vi "8-Axis Roadshow Demo WPC-IPAD.vi"() -> ()   [LabVIEW 2014]
uses:
  Typedef/Typedef_Motor_Message.ctl
  EMC API/EMC_Typedef_Motor_Parameters.ctl
  Functional_Global/Typedef_Message_Queue_Action.ctl
  Functional_Global/Typedef_FPGA_Interface_Action.ctl
  Globals/Global Stop.vi
  Globals/Default Motor Parameters.vi
  <vilib>/Motion/Express/_s/nimc.ex.clearFaults.clearFaults.axis.vi
  <vilib>/Motion/Express/_s/nimc.ex.power.power.axis.vi
  <vilib>/Motion/Express/_s/nimc.ex.resetPosition.resetPosition.axis.vi
  <vilib>/Motion/Express/_s/nimc.ex.read.readTrajectoryData.axis.vi
  <vilib>/Motion/BlockNode/FB.NIMotion.xnode
  support/Message Queue/Message Queue.lvlib
  <vilib>/NI_Real-Time Target Support.lvlib
panel:
  in  "Mode":u16
  in  "# whole revs":dbl=3.0 format="%#_13g"
  in  "Stop all motors":bool
  in  "Max delay (ms)":u32=1000
  in  "Motion Parameters (Min)":T1={"position"=-2000.0, "velocity"=500.0, "acceleration"=5000.0, "deceleration"=5000.0, "accel. jerk"=80000.0, "decel. jerk"=80000.0}
  in  "Motion Parameters (Max)":T1={"position"=2000.0, "velocity"=1500.0, "acceleration"=10000.0, "deceleration"=10000.0, "accel. jerk"=100000.0, "decel. jerk"=100000.0}
  in  "Command Array":string[](array[string])=["ABS Pos Move", "REL Pos Move", "Velocity Move"]
  out "Command":T2={"Axis"="Axis 8", "Motion Parameters"={"position"=0.0, "velocity"=0.0, "acceleration"=0.0, "deceleration"=0.0, "accel. jerk"=0.0, "decel. jerk"=0.0}}
  out "Message":string="Stop"
  out "# elements in queue":i32=9
  out "error out":errorcluster
  out "Axis Positions":T3(graph)={"[0]"=16540.00000000011, "[1]"=7939.956878279383, "[2]"=-7459.9999999999345, "[3]"=-3059.9999999999545, "[4]"=-26059.999999999975, "[5]"=22740.000000000004, "[6]"=3139.9999999999973, "[7]"=11139.999999999998}
  out "Axis Velocities":T3(graph)
  out "Array":dbl[](array[knob])=[140.00000000010914, 139.9568782793831, 140.00000000006548, 140.00000000004547, 140.00000000002547, 140.00000000000364, 139.99999999999727, 139.99999999999818] scale=0.0..200.0
  in  "stop":bool
  # "This example demonstrates how to set up an multi-axis SW architecture using SoftMotion.  You can have state machines that \"produce\" the motion commands, and the consumer will then digest them one at a time.\n\nIn this example, 3 producer loops generate random motion commands at random times (within 1000ms each iteration.) This VI is also meant as a stress test to see if the SM engine is robust enough for complex sequences of motion commands."
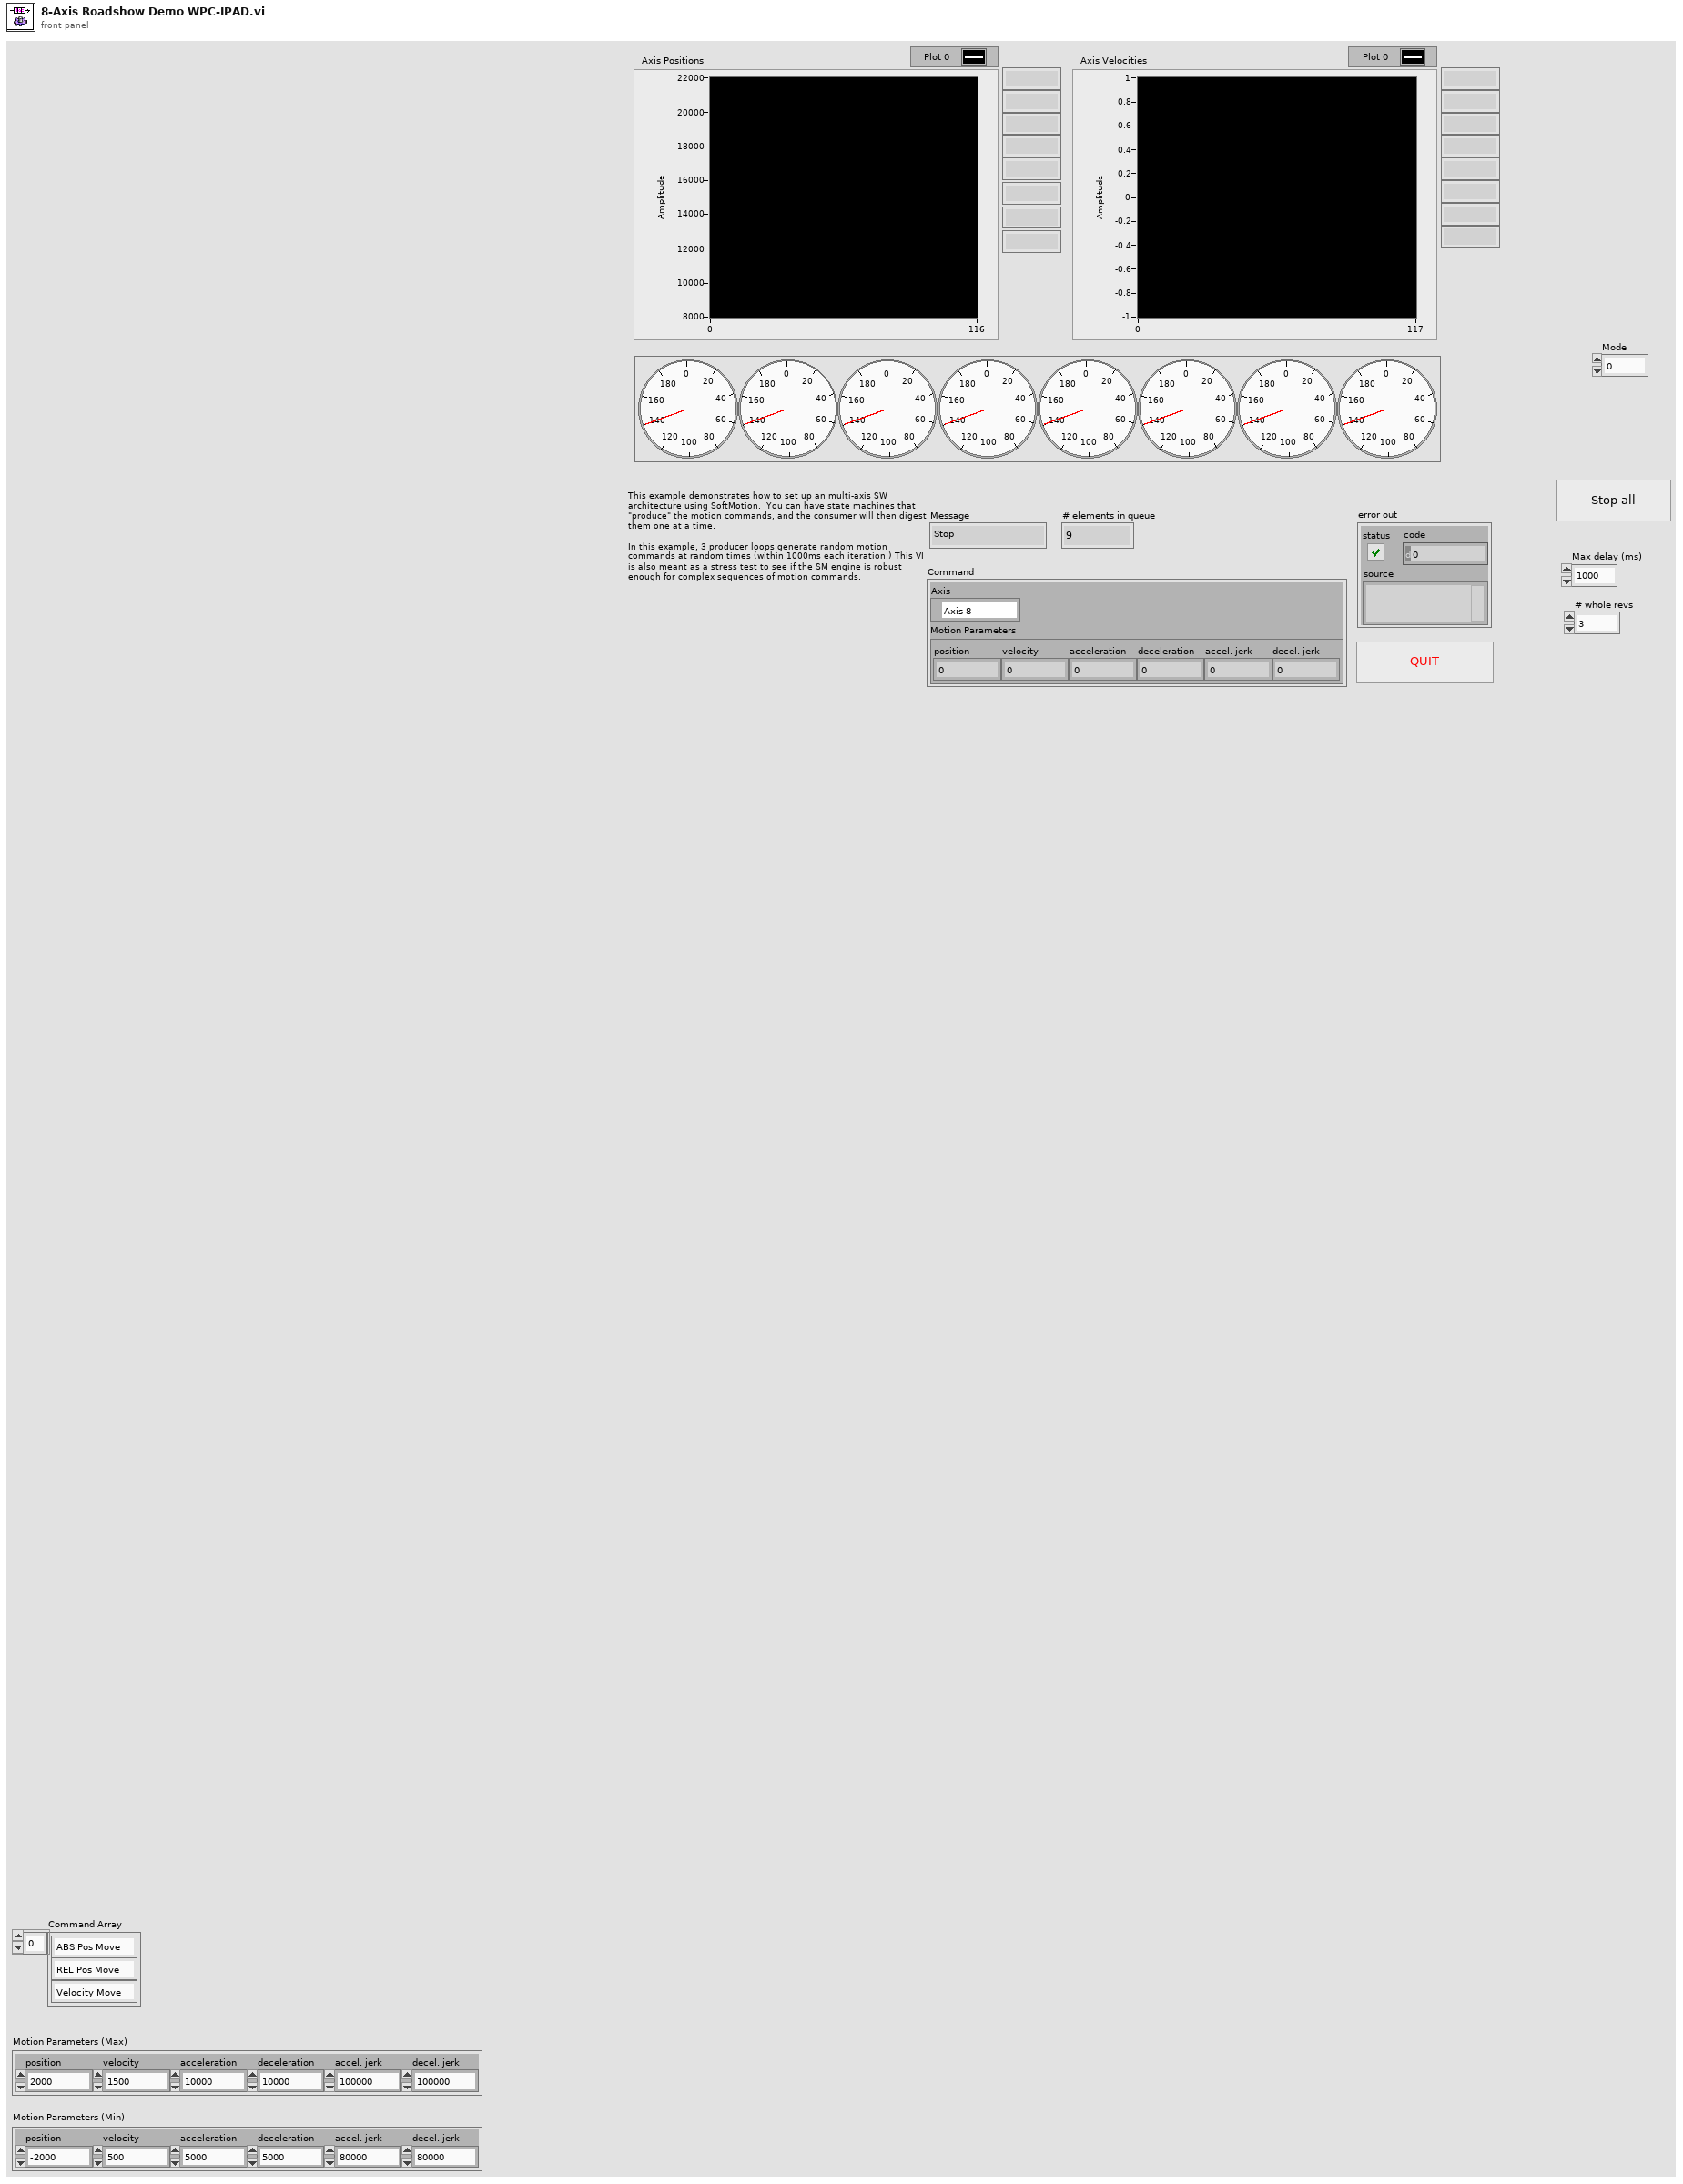
[diagram p1: front panel]
types:
  T1 = typedef "EMC_Typedef_Motor_Parameters.ctl" = cluster{"position":dbl, "velocity":dbl, "acceleration":dbl, "deceleration":dbl, "accel. jerk":dbl, "decel. jerk":dbl}
  T2 = typedef "Typedef_Motor_Message.ctl" = cluster{"Axis":refnum<k21>, "Motion Parameters":T1}
  T3 = cluster{"[0]":dbl, "[1]":dbl, "[2]":dbl, "[3]":dbl, "[4]":dbl, "[5]":dbl, "[6]":dbl, "[7]":dbl}
  T4 = typedef "Typedef_Message_Queue_Action.ctl" = enum16{"Init MQueue", "Get MQueue Ref", "Close MQueue"}
  T5 = typedef "Typedef_FPGA_Interface_Action.ctl" = enum16{"Initialize FPGA", "Get FPGA Reference", "Close FPGA"}
  T6 = typedef "Message Queue.lvlib/Message Cluster.ctl" = cluster{"Message":string, "Message Data":variant}
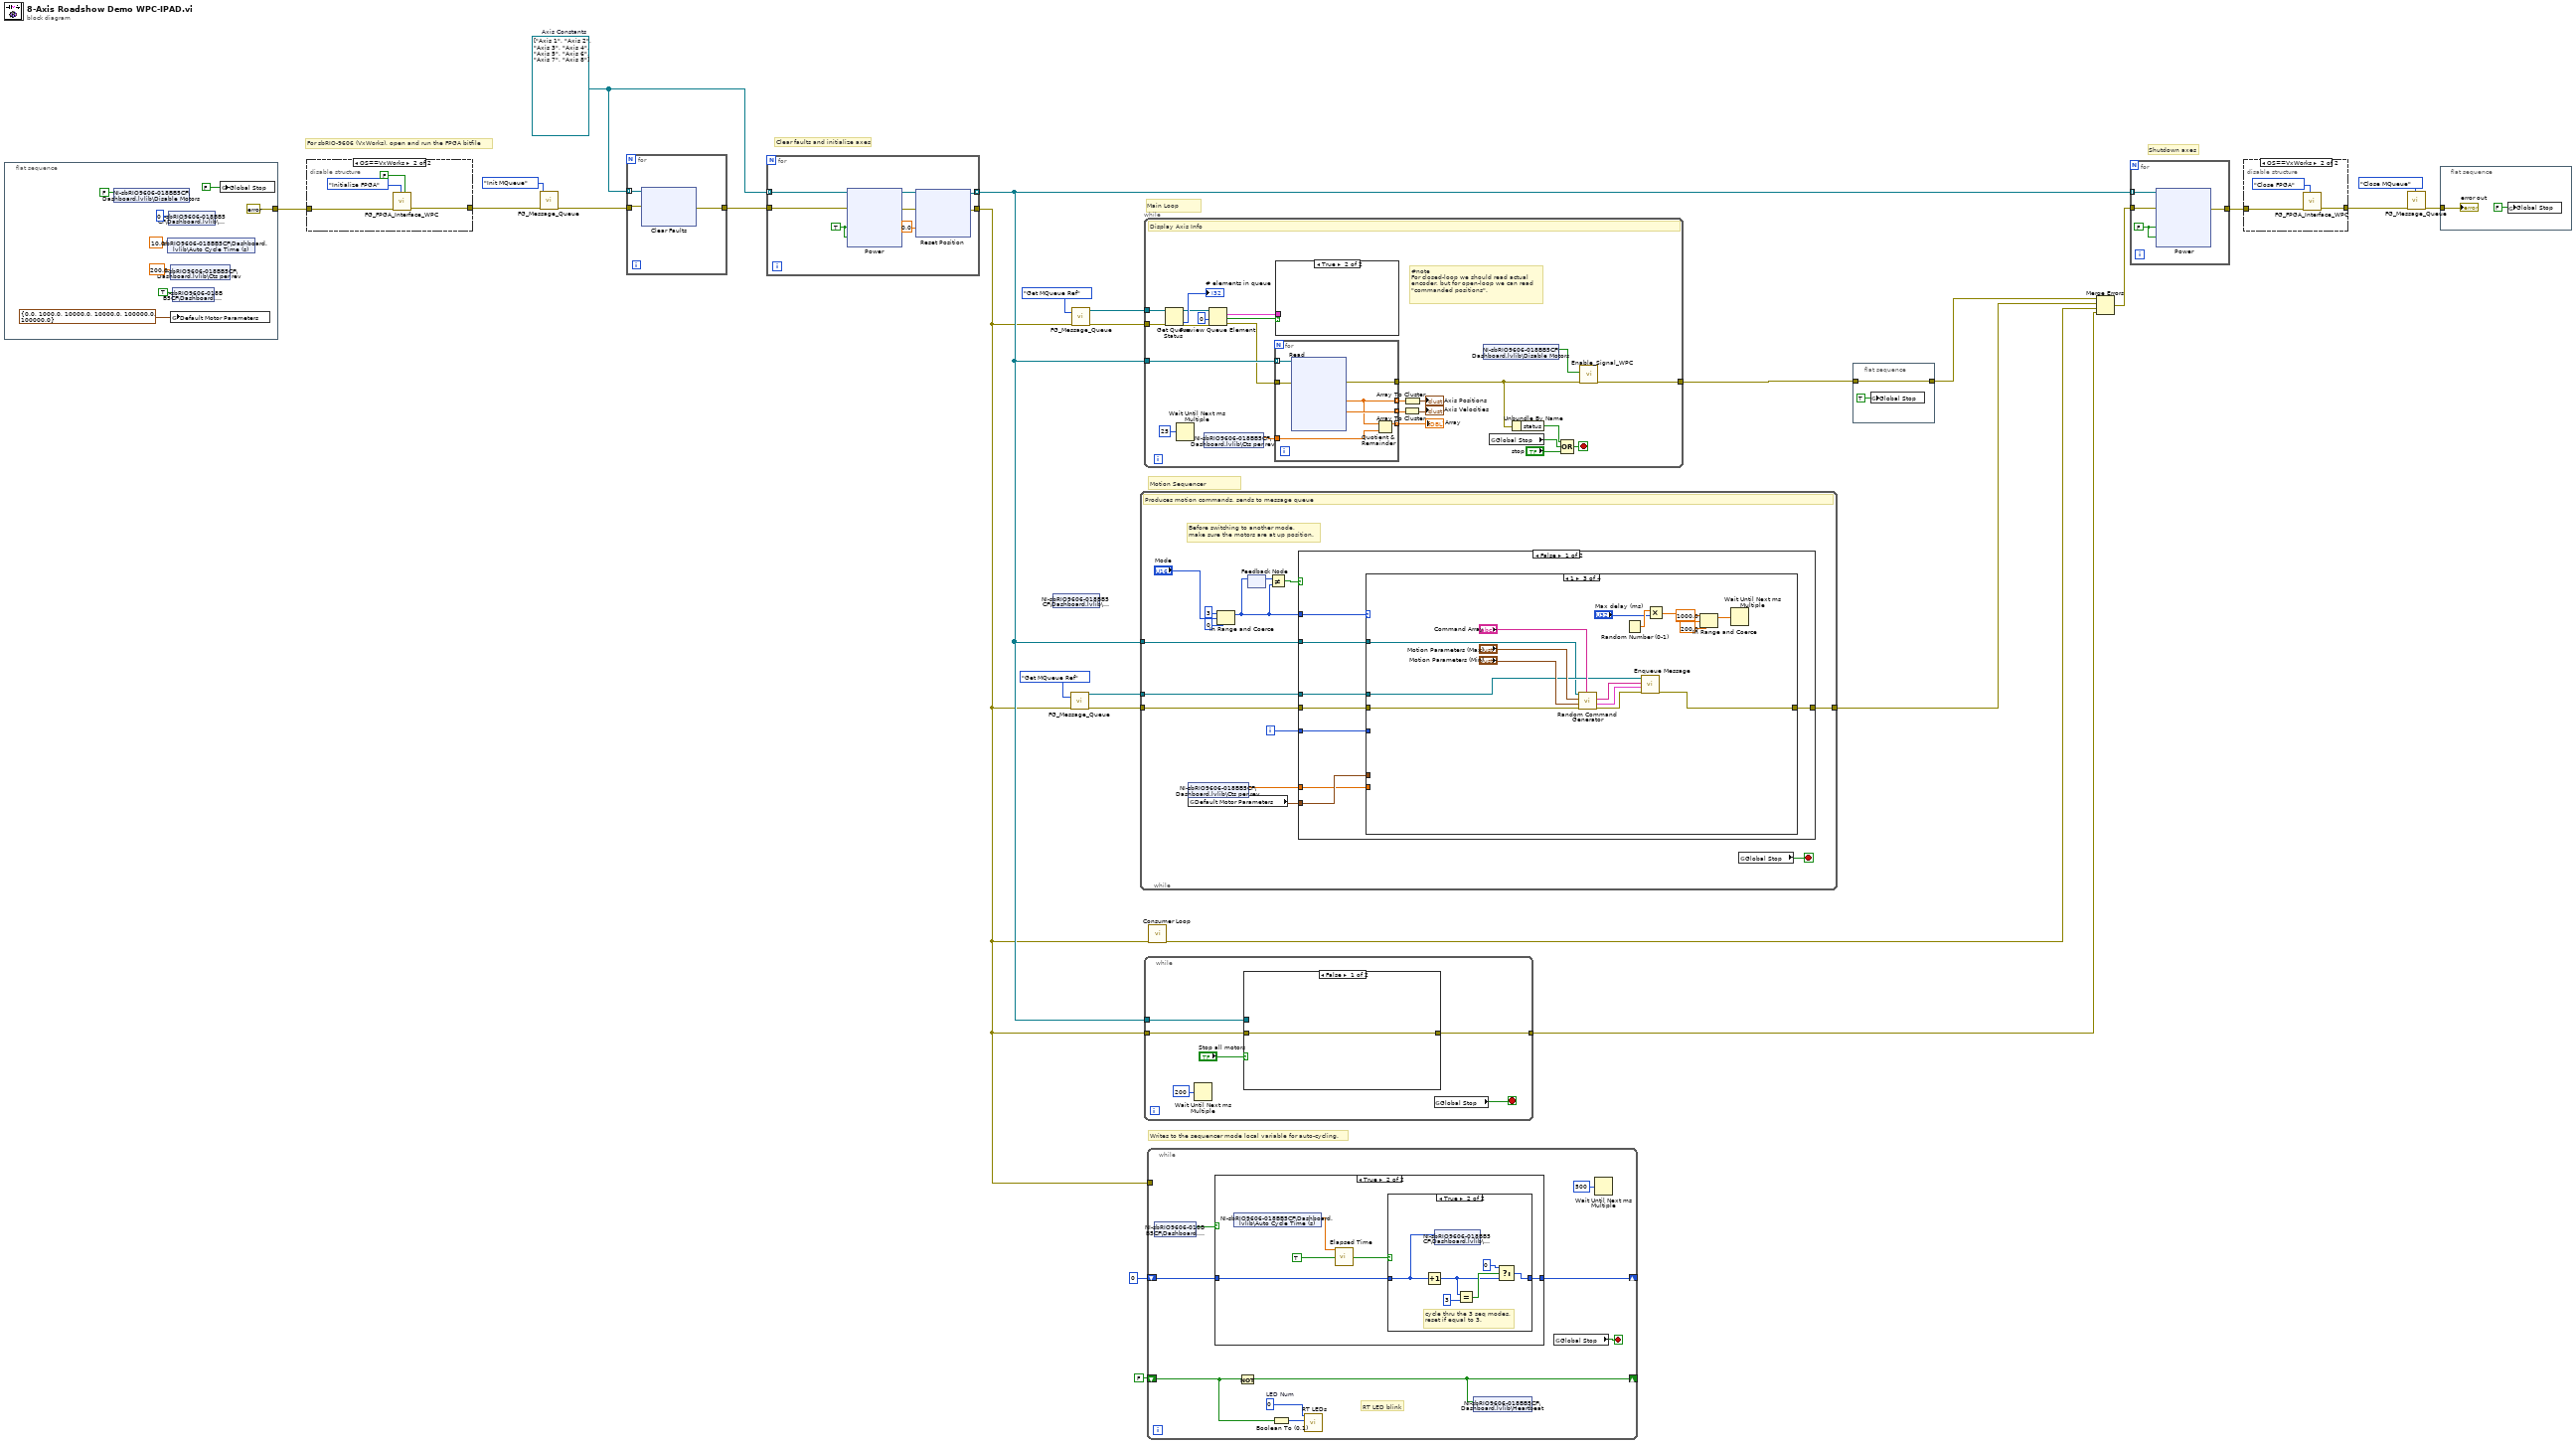
[diagram p0: block diagram]
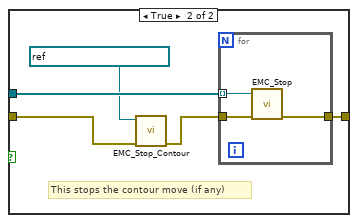
[diagram p4: hidden frame]
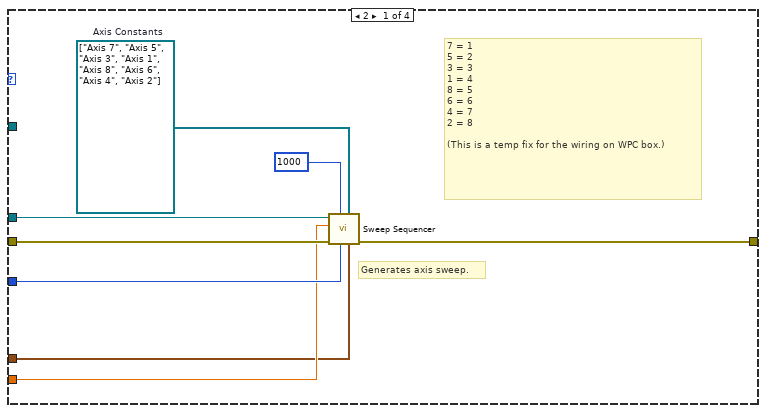
[diagram p5: hidden frame]
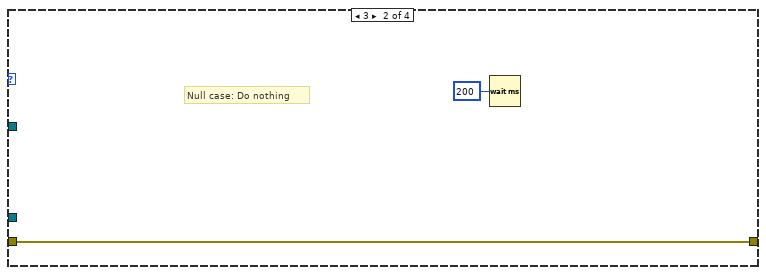
[diagram p6: hidden frame]
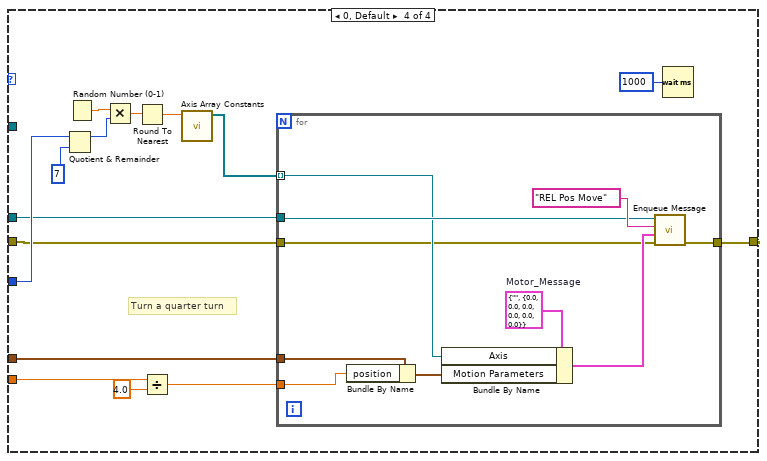
[diagram p7: hidden frame]
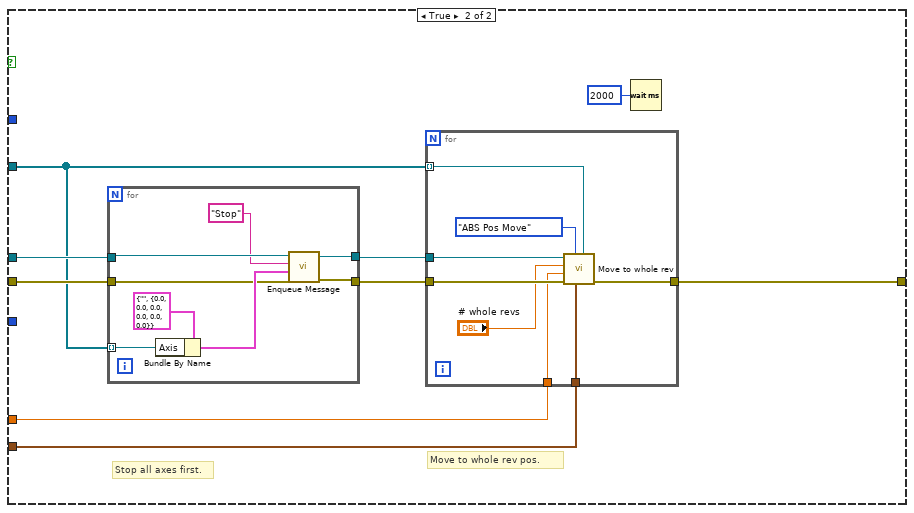
[diagram p8: hidden frame]
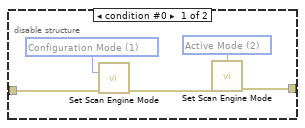
[diagram p10: hidden frame]
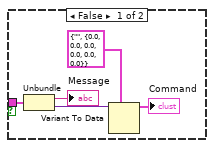
[diagram p11: hidden frame]
diagram:
  w1 = refnum<k21>[] ["Axis 1", "Axis 2", "Axis 3", "Axis 4", "Axis 5", "Axis 6", "Axis 7", "Axis 8"]  # Axis Constants
  # "Writes to the sequencer mode local variable for auto-cycling."
  # "Motion Sequencer"
  # "For sbRIO-9606 (VxWorks), open and run the FPGA bitfile"
  # "Shutdown axes"
  # "Main Loop"
  # "Clear faults and initialize axes"
  n1 = flat-sequence {
    tunnel: [errorcluster {"status"=FALSE, "code"=0, "source"=""} ("error in (no error)")] -> w26
    frame #0 {
      n2 = shared-variable "NI-sbRIO9606-018BB5CF\\Dashboard.lvlib\\Disable Motors"(FALSE ("Disable Motors")) -> ()  [unwired: 1 in, 1 out]
      n3 = shared-variable "NI-sbRIO9606-018BB5CF\\Dashboard.lvlib\\Auto Cycle Time (s)"(10.0 ("Auto Cycle Time (s)")) -> ()  [unwired: 1 in, 1 out]
      n4 = shared-variable "NI-sbRIO9606-018BB5CF\\Dashboard.lvlib\\Mode"(u16 0 ("Mode")) -> ()  [unwired: 1 in, 1 out]
      n5 = shared-variable "NI-sbRIO9606-018BB5CF\\Dashboard.lvlib\\Cts per rev"(200.0 ("Cts per rev")) -> ()  [unwired: 1 in, 1 out]
      n6 = global write "Default Motor Parameters.vi" "Default Motor Parameters"(T1 {"position"=0.0, "velocity"=1000.0, "acceleration"=10000.0, "deceleration"=10000.0, "accel. jerk"=100000.0, "decel. jerk"=100000.0} ("Default Motor Parameters")) -> ()
      n7 = shared-variable "NI-sbRIO9606-018BB5CF\\Dashboard.lvlib\\Auto"(TRUE ("Auto")) -> ()  [unwired: 1 in, 1 out]
      n8 = global write "Global Stop.vi" "Global Stop"(FALSE ("stop")) -> ()
    }
  }
  n9 = disable-structure shown="OS==VxWorks" {
    disable-tunnel: [w39 w41] -> w22
    disable-tunnel: w26 -> [w38 w42]
    frame condition #0 {
      w35 = 1 items=["Configuration Mode"=1, "Active Mode"=2] ("mode (Active Mode)")
      w36 = 2 items=["Configuration Mode"=1, "Active Mode"=2] ("mode (Active Mode)")
      n10 = call <vilib>:"Set Scan Engine Mode.vi"("mode (Active Mode)"=w35, "error in (no error)"=w38) -> ("error out"=w37:errorcluster)  [unwired: 13 in]
      n11 = call <vilib>:"Set Scan Engine Mode.vi"("mode (Active Mode)"=w36, "error in (no error)"=w37) -> ("error out"=w39:errorcluster)  [unwired: 13 in]
    }
    frame condition #1 (active) {
      n12 = call "FG_FPGA_Interface_WPC.vi"("Invert Dir?"=FALSE, "Action"=Typedef_FPGA_Interface_Action."Initialize FPGA", "error in"=w42) -> ("error out"=w41:errorcluster)  [unwired: 7 in, 1 out]
    }
  }
  n13 = call "FG_Message_Queue.vi"("Action"=Typedef_Message_Queue_Action."Init MQueue", "error in"=w22) -> ("error out"=w3:errorcluster)  [unwired: 8 in, 1 out]
  n14 = for {
    tunnel: w3 -> [w46]
    tunnel: [w45] -> w2
    tunnel: w1 -> [w44] mode=indexing
    n15 = xnode ("Clear Faults")("resource"=w44, "error in"=w46) -> ("error out"=w45:errorcluster)  [unwired: 1 out]
  }
  n16 = for {
    tunnel: [w55] -> w6
    tunnel: [w53] -> w8 mode=indexing
    tunnel: w2 -> [w52]
    tunnel: w1 -> [w51] mode=indexing
    w58 = TRUE ("enable axis")
    n17 = xnode ("Power")("enable axis"=w58, "enable drive"=w58, "resource"=w51, "error in"=w52) -> ("resource out"=w54:refnum<k21>, "error out"=w56:errorcluster)
    n18 = xnode ("Reset Position")("position"=0.0, "resource"=w54, "error in"=w56) -> ("resource out"=w53:refnum<k21>, "error out"=w55:errorcluster)
  }
  n19 = shared-variable "NI-sbRIO9606-018BB5CF\\Dashboard.lvlib\\Mode"() -> ()  [unwired: 1 in, 2 out]
  n20 = call "FG_Message_Queue.vi"("Action"=Typedef_Message_Queue_Action."Get MQueue Ref", "error in"=w6) -> ("error out"=w11:errorcluster, "Message Queue"=w10:refnum<queue>)  [unwired: 8 in]
  n21 = call "FG_Message_Queue.vi"("Action"=Typedef_Message_Queue_Action."Get MQueue Ref", "error in"=w6) -> ("error out"=w14:errorcluster, "Message Queue"=w15:refnum<queue>)  [unwired: 8 in]
  n22 = while {
    tunnel: w8 -> [w84]
    tunnel: w11 -> [w86]
    tunnel: w10 -> [w85]
    tunnel: [w82] -> w9
    i -> [w83]
    stop <- w87 stop-if-true
    # "Before switching to another mode,\nmake sure the motors are at up position."
    # "Produces motion commands, sends to message queue"
    n23 = shared-variable "NI-sbRIO9606-018BB5CF\\Dashboard.lvlib\\Cts per rev"() -> (w75:dbl)  [unwired: 1 in, 1 out]
    n24 = global read "Default Motor Parameters.vi" "Default Motor Parameters"() -> (w79:T1)
    n25 = In Range and Coerce(upper limit=u16 3, x="Mode", lower limit=u16 0) -> (coerced(x)=w76:u16)  [unwired: 1 out]
    n26 = feedback-in #1(w76) -> ()
    n27 = feedback #1() -> (w81:u16)  [unwired: 1 in]
    n28 = Not Equal?(x=w81, y=w76) -> (x != y?=w80:bool)
    n29 = case shown="False" w80 {
      tunnel: w86 -> [w95 w152]
      tunnel: w85 -> [w94 w153]
      tunnel: w84 -> [w93 w149]
      tunnel: w83 -> [w92 _]
      tunnel: [w91 w155] -> w82
      tunnel: w76 -> [w90 _]
      tunnel: w79 -> [w89 w148]
      tunnel: w75 -> [w88 w147]
      frame False {
        n30 = case shown="1" w90 {
          tunnel: w95 -> [w103 w105 w115 w134]
          tunnel: w94 -> [w101 _ w114 w132]
          tunnel: w93 -> [_ _ w113 _]
          tunnel: w92 -> [w102 _ _ w135]
          tunnel: [w100 w105 w111 w133] -> w91
          tunnel: w89 -> [w97 _ _ w127]
          tunnel: w88 -> [w98 _ _ w126]
          frame 2 {
            w96 = refnum<k21>[] ["Axis 7", "Axis 5", "Axis 3", "Axis 1", "Axis 8", "Axis 6", "Axis 4", "Axis 2"]  # Axis Constants
            # "7 = 1\n5 = 2\n3 = 3\n1 = 4\n8 = 5\n6 = 6\n4 = 7\n2 = 8\n\n(This is a temp fix for the wiring on WPC box.)"
            # "Generates axis sweep."
            n31 = call "Sweep Sequencer.vi"("Default Motor Parameters"=w97, "Axis Array"=w96, "Loop counter in"=w102, "Max delay (ms)"=u32 1000, "error in (no error)"=w103, "cts per rev"=w98, "Message Queue"=w101) -> ("error out"=w100:errorcluster)  [unwired: 4 in]
          }
          frame 3 {
            # "Null case: Do nothing"
            n32 = Wait (ms)(milliseconds to wait=u32 200) -> ()  [unwired: 1 out]
          }
          frame 1 {
            n33 = call "Random Command Generator.vi"("Command Array"="Command Array", "error in (no error)"=w115, "Motion Parameters (Min)"="Motion Parameters (Min)", "Motion Parameters (Max)"="Motion Parameters (Max)", "Axis Resources"=w113) -> ("error out"=w116:errorcluster, "Motor_Message"=w118:T2, "Command Out"=w117:string)  [unwired: 4 in]
            n34 = Random Number (0-1)() -> (number: 0 to 1=w112:dbl)
            n35 = call "Enqueue Message.vi"("error in (no error)"=w116, "Message Data"=w118, "Message"=w117, "Message Queue"=w114) -> ("error out"=w111:errorcluster)  [unwired: 6 in, 1 out]
            n36 = Multiply(x=w112, y="Max delay (ms)") -> (x*y=w109:dbl)
            n37 = In Range and Coerce(upper limit=1000.0, x=w109, lower limit=200.0) -> (coerced(x)=w106:dbl)  [unwired: 1 out]
            n38 = Wait Until Next ms Multiple(millisecond multiple=w106) -> ()  [unwired: 1 out]
          }
          frame 0, Default {
            # "Turn a quarter turn"
            n39 = Quotient & Remainder(x=w135, y=7) -> (x-y*floor(x/y)=w129:i32)  [unwired: 1 out]
            n40 = Random Number (0-1)() -> (number: 0 to 1=w130:dbl)
            n41 = Multiply(x=w130, y=w129) -> (x*y=w128:dbl)
            n42 = Round To Nearest(number=w128) -> (nearest integer value=w122:dbl)
            n43 = Divide(x=w126, y=4.0) -> (x/y=w124:dbl)
            n44 = call "Axis Array Constants.vi"("Numeric"=w122) -> ("Axis Constants"=w123:refnum<k21>[])  [unwired: 10 in]
            n45 = for {
              tunnel: w123 -> [w141] mode=indexing
              tunnel: w134 -> [w140]
              tunnel: [w139] -> w133
              tunnel: w124 -> [w142]
              tunnel: w132 -> [w143]
              tunnel: w127 -> [w137]
              w146 = T2 {"Axis"="", "Motion Parameters"={"position"=0.0, "velocity"=0.0, "acceleration"=0.0, "deceleration"=0.0, "accel. jerk"=0.0, "decel. jerk"=0.0}}  # Motor_Message
              n46 = Bundle By Name(cluster=w137, "position"=w142) -> (w138:T1)
              n47 = Bundle By Name(cluster=w146, "Axis"=w141, "Motion Parameters"=w138) -> (w145:T2)
              n48 = call "Enqueue Message.vi"("error in (no error)"=w140, "Message Data"=w145, "Message"="REL Pos Move", "Message Queue"=w143) -> ("error out"=w139:errorcluster)  [unwired: 6 in, 1 out]
            }
            n49 = Wait (ms)(milliseconds to wait=u32 1000) -> ()  [unwired: 1 out]
          }
        }
      }
      frame True {
        # "Move to whole rev pos."
        # "Stop all axes first."
        n50 = for {
          tunnel: w153 -> [w163]
          tunnel: w152 -> [w157]
          tunnel: [w156] -> w151
          tunnel: [w161] -> w150
          tunnel: w149 -> [w158] mode=indexing
          n51 = Bundle By Name(cluster=T2 {"Axis"="", "Motion Parameters"={"position"=0.0, "velocity"=0.0, "acceleration"=0.0, "deceleration"=0.0, "accel. jerk"=0.0, "decel. jerk"=0.0}} ("Motor_Message"), "Axis"=w158) -> (w159:T2)
          n52 = call "Enqueue Message.vi"("error in (no error)"=w157, "Message Data"=w159, "Message"="Stop", "Message Queue"=w163) -> ("error out"=w156:errorcluster, "dup Message Queue"=w161:refnum<queue>)  [unwired: 6 in]
        }
        n53 = for {
          tunnel: w149 -> [w167] mode=indexing
          tunnel: w151 -> [w171]
          tunnel: [w170] -> w155
          tunnel: w150 -> [w169]
          tunnel: w148 -> [w166]
          tunnel: w147 -> [w165]
          n54 = call "Move to whole rev.vi"("resource in"=w167, "Default Motor Parameters"=w166, "Mode"=enum16{"ABS Pos Move", "REL Pos Move"}."ABS Pos Move", "error in (no error)"=w171, "cts per rev"=w165, "# whole revs"="# whole revs", "Queue in"=w169) -> ("error out"=w170:errorcluster)  [unwired: 3 in, 1 out]
        }
        n55 = Wait (ms)(milliseconds to wait=u32 2000) -> ()  [unwired: 1 out]
      }
    }
    n56 = global read "Global Stop.vi" "Global Stop"() -> (w87:bool)
  }
  n57 = while {
    tunnel: w14 -> [w184]
    tunnel: w8 -> [w193]
    tunnel: [w173] -> w24
    tunnel: w15 -> [w186]
    stop <- w187 stop-if-true
    # "#note \nFor closed-loop we should read actual \nencoder, but for open-loop we can read\n\"commanded positions\"."
    # "Display Axis Info"
    n58 = Get Queue Status(queue=w186, error in (no error)=w184) -> (queue out=w180:refnum<queue>, error out=w182:errorcluster, # elements in queue=→"# elements in queue":i32)  [unwired: 1 in, 5 out]
    n59 = Wait Until Next ms Multiple(millisecond multiple=u32 25) -> ()  [unwired: 1 out]
    n60 = shared-variable "NI-sbRIO9606-018BB5CF\\Dashboard.lvlib\\Cts per rev"() -> (w177:dbl)  [unwired: 1 in, 1 out]
    n61 = Preview Queue Element(queue=w180, timeout in ms (-1)=0, error in (no error)=w182) -> (element=w179:T6, timed out?=w178:bool, error out=w181:errorcluster)  [unwired: 1 out]
    n62 = for {
      tunnel: [w207] -> w174
      tunnel: [w203] -> w176 mode=indexing
      tunnel: [w206] -> w175 mode=indexing
      tunnel: w181 -> [w205]
      tunnel: w193 -> [w204] mode=indexing
      tunnel: [w202] -> w192 mode=indexing
      tunnel: w177 -> [w201]
      n63 = xnode ("Read")("resource"=w204, "error in"=w205) -> ("commanded position"=w203:dbl, "commanded vel."=w206:dbl, "error out"=w207:errorcluster)  [unwired: 2 out]
      n64 = Quotient & Remainder(x=w203, y=w201) -> (x-y*floor(x/y)=w202:dbl)  [unwired: 1 out]
    }
    "Array" <- w192
    n65 = case shown="True" w178 {
      tunnel: w179 -> [w200 _]
      frame False {
        n66 = Unbundle(w200) -> ("Message"=→"Message":string, "Message Data"=w197:variant)
        n67 = Variant To Data(type=T2 {"Axis"="", "Motion Parameters"={"position"=0.0, "velocity"=0.0, "acceleration"=0.0, "deceleration"=0.0, "accel. jerk"=0.0, "decel. jerk"=0.0}} ("Motor_Message"), Variant=w197) -> (data=→"Command":T2)  [unwired: 1 in, 1 out]
      }
      frame True {
      }
    }
    n68 = Array To Cluster(array=w175) -> (cluster=→"Axis Velocities":T3)
    n69 = Array To Cluster(array=w176) -> (cluster=→"Axis Positions":T3)
    n70 = shared-variable "NI-sbRIO9606-018BB5CF\\Dashboard.lvlib\\Disable Motors"() -> (w172:bool)  [unwired: 1 in, 1 out]
    n71 = global read "Global Stop.vi" "Global Stop"() -> (w188:bool)
    n72 = Unbundle By Name(w174) -> ("status"=w189:bool)
    n73 = Compound Arithmetic op=OR(w189, w188, "stop") -> (w187:bool)
    n74 = call "Enable_Signal_WPC.vi"("error in (no error)"=w174, "Enable (active low)"=w172) -> ("error out"=w173:errorcluster)  [unwired: 9 in]
  }
  n75 = while {
    tunnel: w6 -> [w220]
    tunnel: w8 -> [w218]
    tunnel: [w217] -> w7
    stop <- w216 stop-if-true
    n76 = Wait Until Next ms Multiple(millisecond multiple=u32 200) -> ()  [unwired: 1 out]
    n77 = case shown="False" "Stop all motors" {
      tunnel: w220 -> [w221 w224]
      tunnel: [w221 w226] -> w217
      tunnel: w218 -> [_ w225]
      frame False {
      }
      frame True {
        # "This stops the contour move (if any)"
        n78 = call "EMC_Stop_Contour.vi"("error in (no error)"=w224, "coordinate"=refnum<k21> "Coordinate Space 1") -> ("error out"=w222:errorcluster)  [unwired: 9 in]
        n79 = for {
          tunnel: w222 -> [w229]
          tunnel: w225 -> [w227] mode=indexing
          tunnel: [w228] -> w226
          n80 = call "EMC_Stop.vi"("error in (no error)"=w229, "axis"=w227) -> ("error out"=w228:errorcluster)  [unwired: 8 in, 1 out]
        }
      }
    }
    n81 = global read "Global Stop.vi" "Global Stop"() -> (w216:bool)
  }
  n82 = while {
    tunnel: w6 -> [_]
    shift-right: [w235] -> _
    shift-left: 0 -> [w236]
    shift-right: [w230] -> _
    shift-left: FALSE -> [w231]
    stop <- w238 stop-if-true
    w233 = 0  # LED Num
    # "RT LED blink"
    n83 = shared-variable "NI-sbRIO9606-018BB5CF\\Dashboard.lvlib\\Auto"() -> (w234:bool)  [unwired: 1 in, 1 out]
    n84 = case shown="True" w234 {
      tunnel: w236 -> [w239 w243]
      tunnel: [w239 w242] -> w235
      frame False {
      }
      frame True {
        n85 = shared-variable "NI-sbRIO9606-018BB5CF\\Dashboard.lvlib\\Auto Cycle Time (s)"() -> (w240:dbl)  [unwired: 1 in, 1 out]
        n86 = call "Elapsed Time"("Time Target (s)"=w240, "Auto Reset"=TRUE) -> ("Time has Elapsed"=w244:bool)  [unwired: 10 in, 7 out]
        n87 = case shown="True" w244 {
          tunnel: w243 -> [w245 w246]
          tunnel: [w245 w247] -> w242
          frame False {
          }
          frame True {
            # "cycle thru the 3 seq modes,\nreset if equal to 3."
            n88 = Increment(x=w246) -> (x+1=w249:i32)
            n89 = shared-variable "NI-sbRIO9606-018BB5CF\\Dashboard.lvlib\\Mode"(w246) -> ()  [unwired: 1 in, 1 out]
            n90 = Equal?(x=w249, y=3) -> (x = y?=w250:bool)
            n91 = Select(t=0, s=w250, f=w249) -> (s? t:f=w247:i32)
          }
        }
      }
    }
    n92 = Not(x=w231) -> (.not. x?=w230:bool)
    n93 = Boolean To (0,1)(Boolean=w231) -> (0, 1=w232:i16)
    n94 = call <vilib>:"RT LEDs.vi"("State"=w232, "LED Num"=w233) -> ()  [unwired: 4 in, 2 out]
    n95 = shared-variable "NI-sbRIO9606-018BB5CF\\Dashboard.lvlib\\Heartbeat"(w230) -> ()  [unwired: 1 in, 1 out]
    n96 = global read "Global Stop.vi" "Global Stop"() -> (w238:bool)
    n97 = Wait Until Next ms Multiple(millisecond multiple=u32 500) -> ()  [unwired: 1 out]
  }
  n98 = call "Consumer Loop.vi"("error in (no error)"=w6) -> ("error out"=w13:errorcluster)  [unwired: 10 in]
  n99 = flat-sequence {
    tunnel: w24 -> [w252]
    tunnel: [w252] -> w17
    frame #0 {
      n100 = global write "Global Stop.vi" "Global Stop"(TRUE ("stop")) -> ()
    }
  }
  n101 = Merge Errors(w17, w9, w13, w7) -> (w21:errorcluster)
  n102 = for {
    tunnel: w8 -> [w257] mode=indexing
    tunnel: [w255] -> w25
    tunnel: w21 -> [w254]
    w256 = FALSE ("enable axis")
    n103 = xnode ("Power")("enable axis"=w256, "enable drive"=w256, "resource"=w257, "error in"=w254) -> ("error out"=w255:errorcluster)  [unwired: 1 out]
  }
  n104 = disable-structure shown="OS==VxWorks" {
    disable-tunnel: [w268 w269] -> w19
    disable-tunnel: w25 -> [w268 w270]
    frame condition #0 {
    }
    frame condition #1 (active) {
      n105 = call "FG_FPGA_Interface_WPC.vi"("Action"=Typedef_FPGA_Interface_Action."Close FPGA", "error in"=w270) -> ("error out"=w269:errorcluster)  [unwired: 8 in, 1 out]
    }
  }
  n106 = call "FG_Message_Queue.vi"("Action"=Typedef_Message_Queue_Action."Close MQueue", "error in"=w19) -> ("error out"=w18:errorcluster)  [unwired: 8 in, 1 out]
  n107 = flat-sequence {
    tunnel: w18 -> [w272]
    frame #0 {
      n108 = global write "Global Stop.vi" "Global Stop"(FALSE ("stop")) -> ()
      "error out" <- w272
    }
  }
